vi "Init.vi"(8 "error in (no error)":errorcluster, 9 "Config File Path":path=path "", 10 "Name":string, 11 "Process In":refnum<class "Process.lvclass">) -> (0 "error out":errorcluster, 3 "Process Out":refnum<class "Process.lvclass">)   [LabVIEW 2020, in "Process.lvclass"]
doc: "Initializes the process and creates necessary references. Anything initialized here is released in the Clear.vi method."
uses:
  Process.lvclass
  Process.lvclass/Process.ctl
  Protected/Broadcasting/Broadcast Message Cluster.ctl
  Base/Base.lvclass
  Public/Lifecycle/Lifecycle State.ctl
  Protected/Messaging/Message Cluster.ctl
  Protected/Messaging/Request Message Cluster.ctl
  <vilib>/Utility/error.llb/Clear Errors.vi
  <vilib>/Utility/error.llb/Error Cluster From Error Code.vi
  <vilib>/ErrorRing/Error Ring.xnode
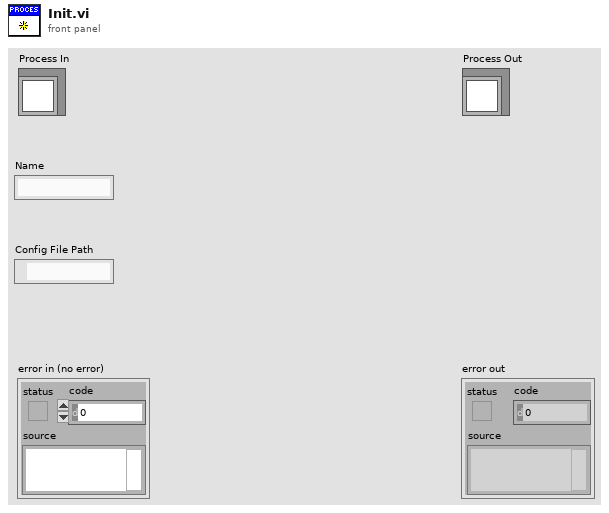
[diagram p1: front panel]
types:
  T1 = typedef "Process.lvclass/Lifecycle State.ctl" = enum16{"Uninitialized", "Initialized", "Started", "Running", "Stopped", "Finished"}
  T2 = typedef "Process.lvclass/Broadcast Message Cluster.ctl" = cluster{"Sender":string, "Message":string, "Message Data":variant}
  T3 = typedef "Process.lvclass/Message Cluster.ctl" = cluster{"Message":string, "Message Data":variant, "Request Notifier":refnum<notifier>}
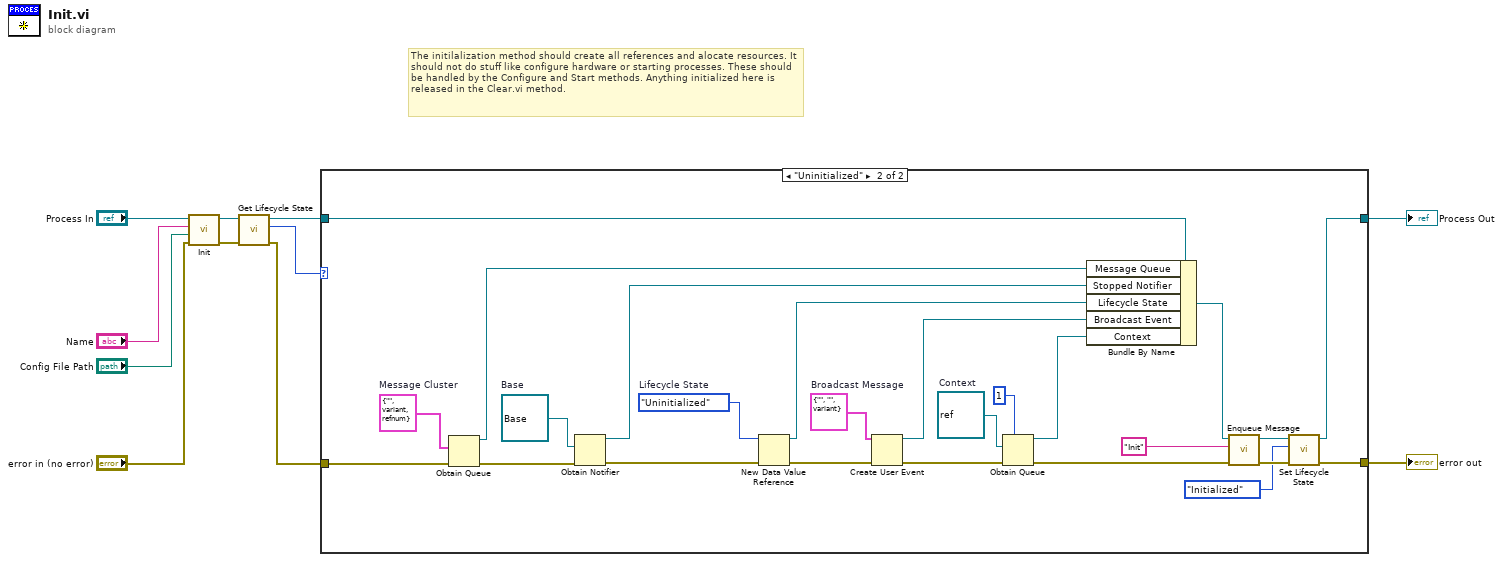
[diagram p0: block diagram]
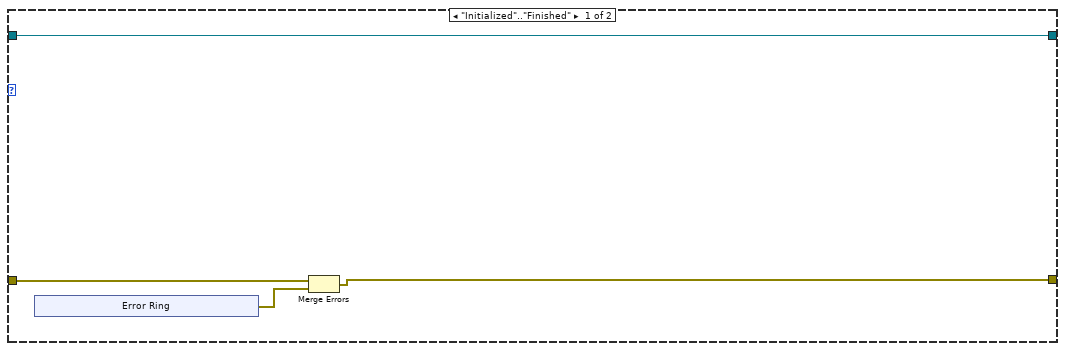
[diagram p2: hidden frame]
diagram:
  # "The initilalization method should create all references and alocate resources. It should not do stuff like configure hardware or starting processes. These should be handled by the Configure and Start methods. Anything initialized here is released in the Clear.vi method."
  n1 = call-parent "Init.vi"("error in (no error)"="error in (no error)", "Config File Path"="Config File Path", "Name"="Name", "Base In"="Process In") -> ("error out"=w2:errorcluster, "Base Out"=w5:refnum<class "Process.lvclass">)  [unwired: 6 in]
  n2 = call "Get Lifecycle State.vi"("error in (no error)"=w2, "Process In"=w5) -> ("error out"=w1:errorcluster, "Lifecycle State"=w10:T1, "Process Out"=w11:refnum<class "Process.lvclass">)  [unwired: 6 in, 1 out]
  n3 = case shown="\"Uninitialized\"" w10 {
    tunnel: [w15 w38] -> w9
    tunnel: [w12 w35] -> w8
    tunnel: w11 -> [w15 w28]
    tunnel: w1 -> [w13 w27]
    frame "Initialized".."Finished" {
      n4 = xnode "Error Ring"() -> ("error out"=w14:errorcluster)
      n5 = Merge Errors(w13, w14) -> (w12:errorcluster)
    }
    frame "Uninitialized" {
      w22 = refnum<class> refnum  # Context
      w26 = T2 {"Sender"="", "Message"="", "Message Data"=variant}  # Broadcast Message
      w30 = refnum<class "Base.lvclass"> refnum  # Base
      w40 = Lifecycle_State."Uninitialized"  # Lifecycle State
      w34 = T3 {"Message"="", "Message Data"=variant, "Request Notifier"=refnum}  # Message Cluster
      n6 = Obtain Queue(element data type=w34, error in (no error)=w27) -> (queue out=w44:refnum<queue>, error out=w33:errorcluster)  [unwired: 3 in, 1 out]
      n7 = Obtain Notifier(notification data type=w30, error in (no error)=w33) -> (notifier out=w29:refnum<notifier>, error out=w41:errorcluster)  [unwired: 2 in, 1 out]
      n8 = New Data Value Reference(data value=w40, error in=w41) -> (data value reference=w39:refnum<data-value>, error out=w31:errorcluster)
      n9 = Create User Event(user event datatype=w26, error in=w31) -> (user event=w25:refnum<user-event>, error out=w24:errorcluster)
      n10 = Obtain Queue(max queue size (-1, unlimited)=1, element data type=w22, error in (no error)=w24) -> (queue out=w20:refnum<queue>, error out=w23:errorcluster)  [unwired: 2 in, 1 out]
      n11 = Bundle By Name(cluster=w28, "Message Queue"=w44, "Stopped Notifier"=w29, "Lifecycle State"=w39, "Broadcast Event"=w25, "Context"=w20) -> (w32:refnum<class "Process.lvclass">)
      n12 = call "Enqueue Message.vi"("error in (no error)"=w23, "Message"="Init", "Process In"=w32) -> ("error out"=w37:errorcluster, "Process Out"=w43:refnum<class "Process.lvclass">)  [unwired: 7 in]
      n13 = call "Set Lifecycle State.vi"("error in (no error)"=w37, "Lifecycle State"=Lifecycle_State."Initialized", "Process In"=w43) -> ("error out"=w35:errorcluster, "Process Out"=w38:refnum<class "Process.lvclass">)  [unwired: 7 in]
    }
  }
  "error out" <- w8
  "Process Out" <- w9
